vi "ABR3-Plot Metrics.vi"(0 "Analysis":T1, 1 "Avg Mode":enum16{"Neural/CM", "ANOW"}(ring), 7 "Plot user metric?":bool, 11 "error in (no error)":errorcluster, 12 "I-O":refnum<vi>) -> (15 "error out":errorcluster)   [LabVIEW 2020]
uses:
  TypeDefs/ABR3-Analysis State.ctl
  Threshold Estimation VIs/ABR3-Threshold Estimation Result.ctl
  <vilib>/Analysis/polynomials.llb/Unique Numbers and Multiplicity (DBL).vi
  epl-vi-lib/Utility VIs/Graphics VIs/Graphics-Sort XY Graph (1D).vi
  <vilib>/Analysis/NI_AALPro.lvlib
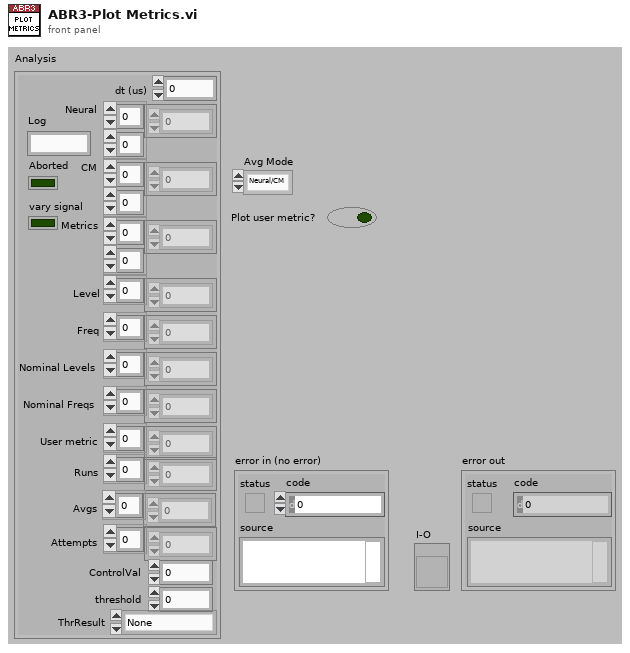
[diagram p1: front panel]
types:
  T1 = typedef "ABR3-Analysis State.ctl" = cluster{"dt (us)":dbl, "Neural":dbl[][], "CM":dbl[][], "Metrics":dbl[][], "Level":dbl[], "Freq":dbl[], "Nominal Levels":dbl[], "Nominal Freqs":dbl[], "User metric":dbl[], "Runs":i32[], "Avgs":i32[], "Attempts":i32[], "Log":string, "Aborted":bool, "ControlVal":dbl, "threshold":dbl, "vary signal":bool, "ThrResult":T2}
  T2 = typedef "ABR3-Threshold Estimation Result.ctl" = enum16{"None", "Power", "Sigmoid", "Power (noisy)", "Suprathreshold", "Invalid"}
  T3 = cluster{"Array Subset":dbl[], "Array Subset":dbl[]}
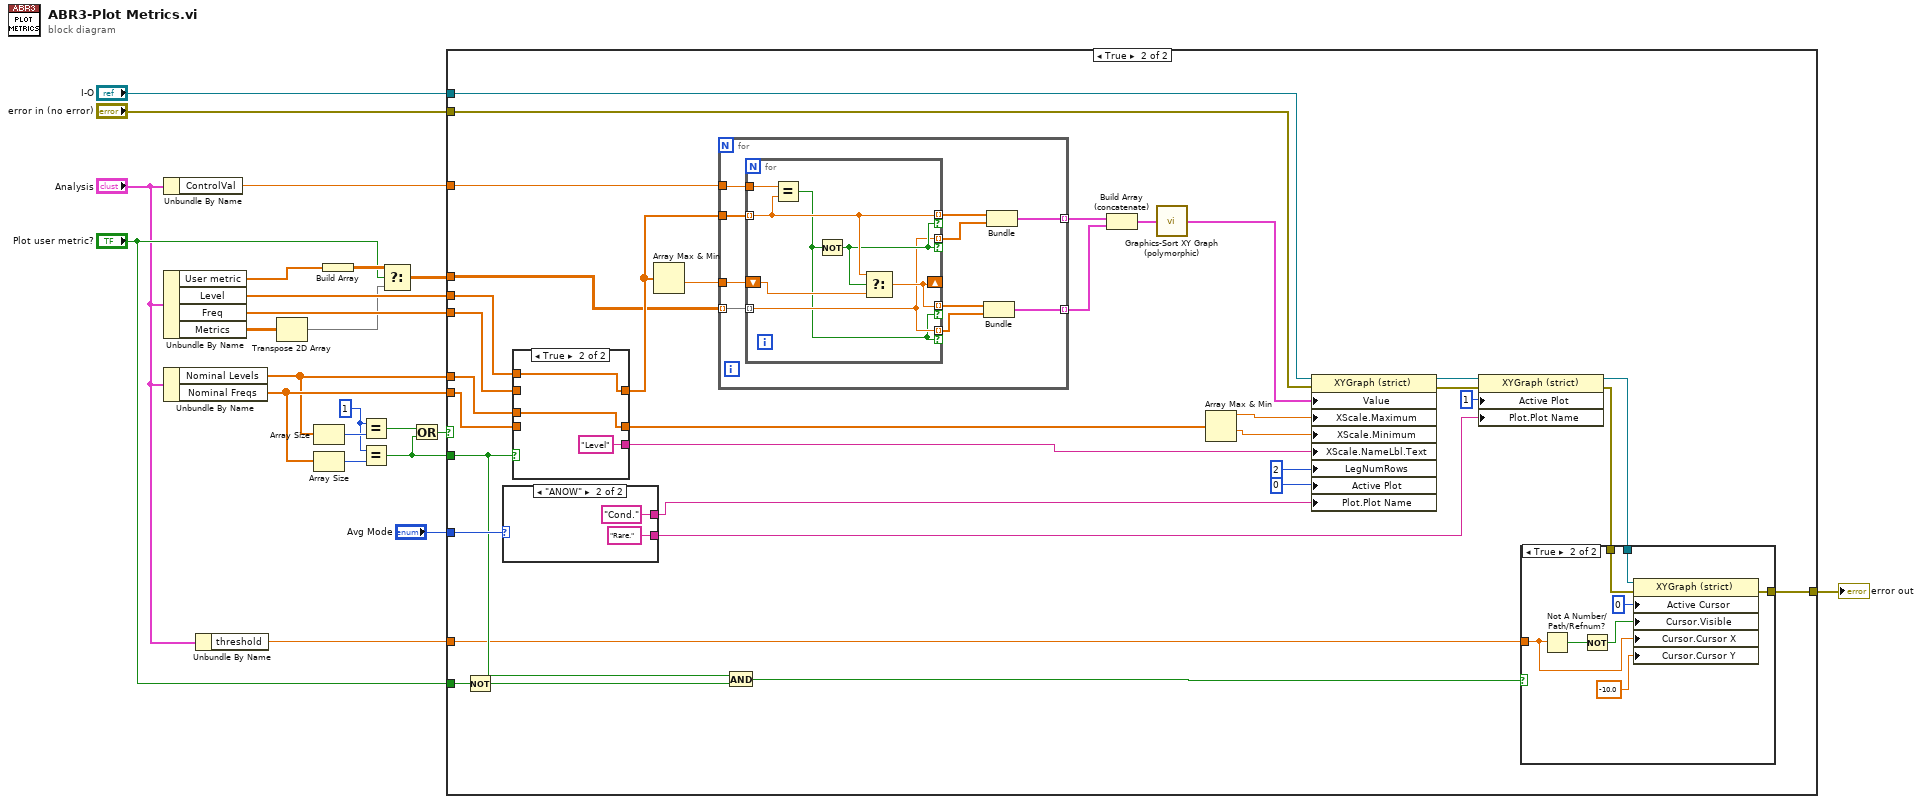
[diagram p0: block diagram]
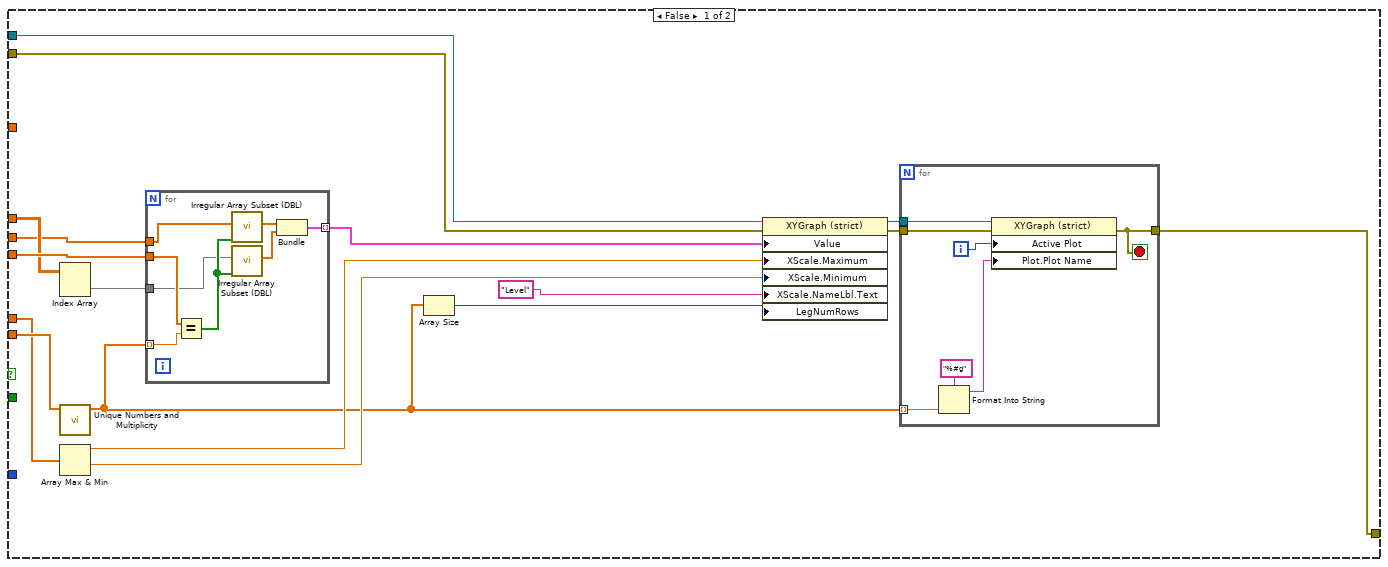
[diagram p2: hidden frame]
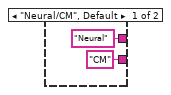
[diagram p4: hidden frame]
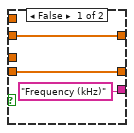
[diagram p5: hidden frame]
diagram:
  w12 = 1
  n1 = Unbundle By Name("Analysis") -> ("ControlVal"=w7:dbl)
  n2 = Unbundle By Name("Analysis") -> ("User metric"=w11:dbl[], "Level"=w15:dbl[], "Freq"=w21:dbl[], "Metrics"=w19:dbl[][])
  n3 = Unbundle By Name("Analysis") -> ("Nominal Levels"=w5:dbl[], "Nominal Freqs"=w6:dbl[])
  n4 = Unbundle By Name("Analysis") -> ("threshold"=w1:dbl)
  n5 = Transpose 2D Array(2D array=w19) -> (transposed array=w4:dbl[][])
  n6 = Array Size(array=w5) -> (size(s)=w23:i32)
  n7 = Array Size(array=w6) -> (size(s)=w18:i32)
  n8 = Build Array(w11) -> (w10:dbl[][])
  n9 = Equal?(x=w12, y=w23) -> (x = y?=w22:bool)
  n10 = Equal?(x=w12, y=w18) -> (x = y?=w16:bool)
  n11 = Select(t=w10, s="Plot user metric?", f=w4) -> (s? t:f=w9:dbl[][])
  n12 = Or(x=w22, y=w16) -> (x .or. y?=w17:bool)
  n13 = case shown="True" w17 {
    tunnel: w21 -> [w39 w78]
    tunnel: "I-O" -> [w34 w60]
    tunnel: "error in (no error)" -> [w35 w87]
    tunnel: w9 -> [w38 w61]
    tunnel: w6 -> [w40 w80]
    tunnel: [w24 w56] -> w14
    tunnel: w16 -> [_ w67]
    tunnel: w5 -> [w32 w79]
    tunnel: w15 -> [w36 w77]
    tunnel: "Avg Mode" -> [_ w76]
    tunnel: w7 -> [_ w70]
    tunnel: "Plot user metric?" -> [_ w66]
    tunnel: w1 -> [_ w63]
    frame False {
      n14 = Index Array(array=w38) -> (element=w37:dbl[])  [unwired: 2 in]
      n15 = call-poly <vilib>:"Unique Numbers and Multiplicity.vi"("Numbers"=w40) -> ("Unique Numbers"=w25:dbl[])  [unwired: 8 in, 2 out]
      n16 = Array Max & Min(array=w32) -> (max value=w31:dbl, min value=w30:dbl)  [unwired: 2 out]
      n17 = for {
        tunnel: w25 -> [w55] mode=indexing
        tunnel: w39 -> [w54]
        tunnel: w37 -> [w52]
        tunnel: w36 -> [w51]
        tunnel: [w48] -> w33 mode=indexing
        n18 = Equal?(x=w54, y=w55) -> (x = y?=w53:bool[])
        n19 = call "Irregular Array Subset (DBL).vi"("Mask"=w53, "Array"=w51) -> ("Array Subset"=w50:dbl[])  [unwired: 8 in, 1 out]
        n20 = call "Irregular Array Subset (DBL).vi"("Mask"=w53, "Array"=w52) -> ("Array Subset"=w49:dbl[])  [unwired: 8 in, 1 out]
        n21 = Bundle("Array Subset"=w50, "Array Subset"=w49) -> (w48:T3)  [unwired: 1 in]
      }
      n22 = Array Size(array=w25) -> (size(s)=w28:i32)
      n23 = property class="XYGraph (strict)"(reference=w34, error in=w35, "Value"=w33, "XScale.Maximum"=w31, "XScale.Minimum"=w30, "XScale.NameLbl.Text"="Level" ("X Scale.Name Label.Text"), "LegNumRows"=w28) -> (reference out=w27:refnum<vi>, error out=w26:errorcluster)
      n24 = for {
        tunnel: w27 -> [w47]
        tunnel: w26 -> [w46]
        tunnel: w25 -> [w43] mode=indexing
        tunnel: [w41] -> w24
        i -> [w45]
        stop <- w41 stop-if-true
        n25 = Format Into String(format string="%#g", w43) -> (resulting string=w42:string)  [unwired: 2 in, 1 out]
        n26 = property class="XYGraph (strict)"(reference=w47, error in=w46, "Active Plot"=w45, "Plot.Plot Name"=w42) -> (error out=w41:errorcluster)  [unwired: 1 out]
      }
    }
    frame True {
      n27 = Not(x=w66) -> (.not. x?=w65:bool)
      n28 = case shown="\"ANOW\"" w76 {
        tunnel: ["Neural" ("Plot.Plot Name") "Cond." ("Plot.Plot Name")] -> w75
        tunnel: ["CM" ("Plot.Plot Name") "Rare." ("Plot.Plot Name")] -> w74
        frame "Neural/CM", Default {
        }
        frame "ANOW" {
        }
      }
      n29 = case shown="True" w67 {
        tunnel: ["Frequency (kHz)" ("X Scale.Name Label.Text") "Level" ("X Scale.Name Label.Text")] -> w81
        tunnel: [w121 w125] -> w59
        tunnel: w80 -> [w121 _]
        tunnel: w79 -> [_ w125]
        tunnel: w78 -> [w120 _]
        tunnel: w77 -> [_ w123]
        tunnel: [w120 w123] -> w62
        frame False {
        }
        frame True {
        }
      }
      n30 = Array Max & Min(array=w62) -> (min value=w71:dbl)  [unwired: 3 out]
      n31 = for {
        tunnel: w70 -> [w108]
        tunnel: w71 -> [w107]
        tunnel: w62 -> [w106]
        tunnel: w61 -> [w105] mode=indexing
        tunnel: [w104] -> w72 mode=indexing
        tunnel: [w101] -> w73 mode=indexing
        n32 = for {
          tunnel: w105 -> [w110] mode=indexing
          tunnel: w108 -> [w115]
          tunnel: w106 -> [w114] mode=indexing
          shift-right: [w112] -> _
          shift-left: w107 -> [w113]
          tunnel: [w110] -> w99 mode=indexing if=w111
          tunnel: [w114] -> w100 mode=indexing if=w111
          tunnel: [w110] -> w103 mode=indexing if=w109
          tunnel: [w112] -> w102 mode=indexing if=w109
          n33 = Equal?(x=w115, y=w114) -> (x = y?=w109:bool)
          n34 = Not(x=w109) -> (.not. x?=w111:bool)
          n35 = Select(t=w114, s=w111, f=w113) -> (s? t:f=w112:dbl)
        }
        n36 = Bundle(w102, w103) -> (w101:cluster{dbl[], dbl[]})  [unwired: 1 in]
        n37 = Bundle(w100, w99) -> (w104:cluster{dbl[], dbl[]})  [unwired: 1 in]
      }
      n38 = And(x=w67, y=w65) -> (x .and. y?=w64:bool)
      n39 = Build Array (concatenate)(w72, w73) -> (w69:cluster{dbl[], dbl[]}[])
      n40 = call-poly "Graphics-Sort XY Graph (polymorphic).vi"("graph"=w69) -> ("sorted graph"=w68:cluster{"x":dbl[], "y":dbl[]}[])  [unwired: 14 in]
      n41 = Array Max & Min(array=w59) -> (max value=w89:dbl, min value=w88:dbl)  [unwired: 2 out]
      n42 = property class="XYGraph (strict)"(reference=w60, error in=w87, "Value"=w68, "XScale.Maximum"=w89, "XScale.Minimum"=w88, "XScale.NameLbl.Text"=w81, "LegNumRows"=u32 2 ("Legend:Number of Rows"), "Active Plot"=u32 0, "Plot.Plot Name"=w75) -> (reference out=w84:refnum<vi>, error out=w83:errorcluster)
      n43 = property class="XYGraph (strict)"(reference=w84, error in=w83, "Active Plot"=u32 1, "Plot.Plot Name"=w74) -> (reference out=w57:refnum<vi>, error out=w58:errorcluster)
      n44 = case shown="True" w64 {
        tunnel: w63 -> [_ w92]
        tunnel: w58 -> [w90 w97]
        tunnel: w57 -> [_ w96]
        tunnel: [w90 w95] -> w56
        frame False {
        }
        frame True {
          n45 = Not A Number/Path/Refnum?(number/path/refnum=w92) -> (NaN/Path/Refnum?=w98:bool)
          n46 = Not(x=w98) -> (.not. x?=w93:bool)
          n47 = property class="XYGraph (strict)"(reference=w96, error in=w97, "Active Cursor"=u32 0, "Cursor.Visible"=w93, "Cursor.Cursor X"=w92, "Cursor.Cursor Y"=-10.0) -> (error out=w95:errorcluster)  [unwired: 1 out]
        }
      }
    }
  }
  "error out" <- w14
